vi "TENMA_Conf_On_P.vi"(8 "errin":errorcluster caption="entrée d'erreur (pas d'erreur)", 10 "Tenma On?":bool, 11 "Visa in tenma":refnum<visa-resource-name>) -> (0 "sortie d'erreur":errorcluster, 3 "VISA resource name out":refnum<visa-resource-name>)   [LabVIEW 2020]
uses:
  <vilib>/Instr/_visa.llb/VISA Configure Serial Port (Instr).vi
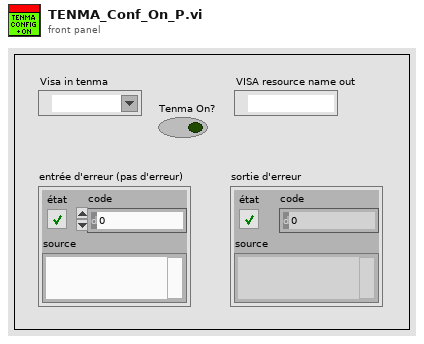
[diagram p1: front panel]
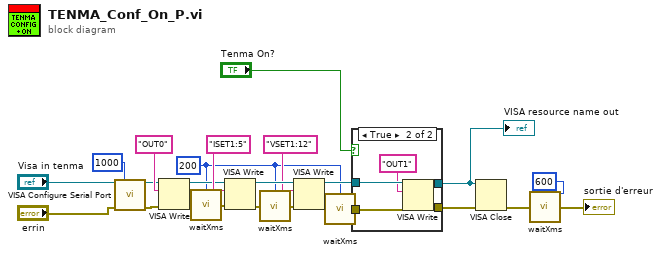
[diagram p0: block diagram]
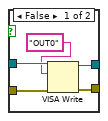
[diagram p2: hidden frame]
diagram:
  w7 = u32 200 ("attente (ms)")
  n1 = call-poly "VISA Configure Serial Port"("VISA resource name"="Visa in tenma", "timeout (10sec)"=u32 1000, "error in (no error)"="errin") -> ("VISA resource name out"=w15:refnum<visa-resource-name>, "error out"=w16:errorcluster)  [unwired: 11 in]
  n2 = VISA Write(VISA resource name=w15, write buffer="OUT0" ("buffer d'écriture"), error in (no error)=w16) -> (VISA resource name out=w14:refnum<visa-resource-name>, error out=w13:errorcluster)  [unwired: 1 out]
  n3 = call <userlib>:"waitXms.vi"("attente (ms)"=w7, "errin"=w13) -> ("errout"=w12:errorcluster)  [unwired: 13 in]
  n4 = VISA Write(VISA resource name=w14, write buffer="ISET1:5" ("buffer d'écriture"), error in (no error)=w12) -> (VISA resource name out=w20:refnum<visa-resource-name>, error out=w11:errorcluster)  [unwired: 1 out]
  n5 = call <userlib>:"waitXms.vi"("attente (ms)"=w7, "errin"=w11) -> ("errout"=w10:errorcluster)  [unwired: 13 in]
  n6 = VISA Write(VISA resource name=w20, write buffer="VSET1:12" ("buffer d'écriture"), error in (no error)=w10) -> (VISA resource name out=w21:refnum<visa-resource-name>, error out=w8:errorcluster)  [unwired: 1 out]
  n7 = call <userlib>:"waitXms.vi"("attente (ms)"=w7, "errin"=w8) -> ("errout"=w9:errorcluster)  [unwired: 13 in]
  n8 = case shown="True" "Tenma On?" {
    tunnel: [w26 w34] -> w24
    tunnel: [w28 w33] -> w23
    tunnel: w21 -> [w27 w32]
    tunnel: w9 -> [w29 w30]
    frame False {
      n9 = VISA Write(VISA resource name=w27, write buffer="OUT0" ("buffer d'écriture"), error in (no error)=w29) -> (VISA resource name out=w26:refnum<visa-resource-name>, error out=w28:errorcluster)  [unwired: 1 out]
    }
    frame True {
      n10 = VISA Write(VISA resource name=w32, write buffer="OUT1" ("buffer d'écriture"), error in (no error)=w30) -> (VISA resource name out=w34:refnum<visa-resource-name>, error out=w33:errorcluster)  [unwired: 1 out]
    }
  }
  "VISA resource name out" <- w24
  n11 = VISA Close(VISA resource name=w24, error in (no error)=w23) -> (error out=w3:errorcluster)
  n12 = call <userlib>:"waitXms.vi"("attente (ms)"=u32 600, "errin"=w3) -> ("errout"=→"sortie d'erreur":errorcluster)  [unwired: 13 in]
